vi "rsscope_core_global.vi"() -> ()   [LabVIEW 2018] (continued)
 parameter.  The trigger does not actually occur until the edge of a pulse that corresponds to the Glitch Width and Glitch Polarity crosses the threshold you specify in the Trigger Level parameter."}, {"Level"=4, "Class Only"=FALSE, "Identifier"="RSSCOPE_ATTR_SEARCH_TRIGGER_GLITCH_ENABLED", "Descriptive Name"="Search Trigger Glitch Enabled", "Data Type"=3, "Command"="SEAR:TRIG:GLIT", "Access"=2, "Range Table"="", "Read Callback"="rsscope_FormatSearchNameBoolean_ReadCallback.vi", "Write Callback"="rsscope_FormatSearchNameBoolean_WriteCallback.vi", "Supported Models"="", "Instrument Options"="", "Flags"=0, "Help"="Includes the search conditions for the glitch trigger event type in the next search.\n\nAvailable Repeated Capabilities:\nNone\n\nRemote-control command(s):\nSEARch:TRIGger:GLITch[:STATe]"}, {"Level"=4, "Class Only"=FALSE, "Identifier"="RSSCOPE_ATTR_SEARCH_TRIGGER_GLITCH_WIDTH", "Descriptive Name"="Search Trigger Glitch Width", "Data Type"=1, "Command"="SEAR:TRIG:GLIT:WIDT", "Access"=2, "Range Table"="RsScope_rngSearchGlitchWidth", "Read Callback"="rsscope_FormatSearchNameReal64_ReadCallback.vi", "Write Callback"="rsscope_FormatSearchNameReal64_WriteCallback.vi", "Supported Models"="", "Instrument Options"="", "Flags"=0, "Help"="Sets the length of a glitch. The instrument triggers on pulses shorter or longer than this value.\n\nAvailable Repeated Capabilities:\nNone\n\nRemote-control command(s):\nSEARch:TRIGger:GLITch:WIDTh"}, {"Level"=4, "Class Only"=FALSE, "Identifier"="RSSCOPE_ATTR_SEARCH_TRIGGER_GLITCH_POLARITY", "Descriptive Name"="Search Trigger Glitch Polarity", "Data Type"=0, "Command"="SEAR:TRIG:GLIT:POL", "Access"=2, "Range Table"="rsscope_rngTriggerSlope", "Read Callback"="rsscope_FormatSearchNameInt32_ReadCallback.vi", "Write Callback"="rsscope_FormatSearchNameInt32_WriteCallback.vi", "Supported Models"="", "Instrument Options"="", "Flags"=0, "Help"="Defines the polarity of a pulse, that is the direction of the first pulse slope.\n\nAvailable Repeated Capabilities:\nNone\n\nRemote-control command(s):\nSEARch:TRIGger:GLITch:POLarity"}, {"Level"=4, "Class Only"=FALSE, "Identifier"="RSSCOPE_ATTR_SEARCH_TRIGGER_GLITCH_CONDITION", "Descriptive Name"="Search Trigger Glitch Condition", "Data Type"=0, "Command"="SEAR:TRIG:GLIT:RANG", "Access"=2, "Range Table"="rsscope_rngWidthCondition", "Read Callback"="rsscope_FormatSearchNameInt32_ReadCallback.vi", "Write Callback"="rsscope_FormatSearchNameInt32_WriteCallback.vi", "Supported Models"="", "Instrument Options"="", "Flags"=0, "Help"="Selects which glitches are identified: shorter or longer than the specified width.\n\nAvailable Repeated Capabilities:\nNone\n\nRemote-control command(s):\nSEARch:TRIGger:GLITch:RANGe"}, {"Level"=4, "Class Only"=FALSE, "Identifier"="RSSCOPE_ATTR_SEARCH_TRIGGER_GLITCH_COPY_FROM_A", "Descriptive Name"="Search Trigger Glitch Copy From A", "Data Type"=4, "Command"="SEAR:TRIG:GLIT:ACOP", "Access"=1, "Range Table"="", "Read Callback"="", "Write Callback"="rsscope_FormatSearchNameEvent_WriteCallback.vi", "Supported Models"="", "Instrument Options"="", "Flags"=0, "Help"="Copies the trigger event configuration from Trigger A for the selected channel source to the search condition settings. Set the selected search name with RSSCOPE_ATTR_SELECTED_SEARCH_NAME.\n\nAvailable Repeated Capabilities:\nNone\n\nRemote-control command(s):\nSEARch:TRIGger:GLITch:ACOPy"}, {"Level"=3, "Class Only"=TRUE, "Identifier"="", "Descriptive Name"="Width", "Data Type"=0, "Command"="", "Access"=0, "Range Table"="", "Read Callback"="", "Write Callback"="", "Supported Models"="", "Instrument Options"="", "Flags"=0, "Help"="Configures the conditions for the width trigger search.  A width trigger occurs when the oscilloscope detects a positive or negative pulse with a width between, or optionally outside, the width thresholds.  You specify the width thresholds with the Width Low Threshold and Width High Threshold parameters.  You specify whether the oscilloscope triggers on pulse widths that are within or outside the width thresholds with the Width Condition parameter.  You specify the polarity of the pulse with the Width Polarity parameter.  The trigger does not actually occur until the edge of a pulse that corresponds to the Width Low Threshold, Width High Threshold, Width Condition, and Width Polarity crosses the threshold you specify in the Trigger Level parameter."}, {"Level"=4, "Class Only"=FALSE, "Identifier"="RSSCOPE_ATTR_SEARCH_TRIGGER_WIDTH_ENABLED", "Descriptive Name"="Search Trigger Width Enabled", "Data Type"=3, "Command"="SEAR:TRIG:WIDT", "Access"=2, "Range Table"="", "Read Callback"="rsscope_FormatSearchNameBoolean_ReadCallback.vi", "Write Callback"="rsscope_FormatSearchNameBoolean_WriteCallback.vi", "Supported Models"="", "Instrument Options"="", "Flags"=0, "Help"="Includes the search conditions for the width trigger event type in the next search.\n\nAvailable Repeated Capabilities:\nNone\n\nRemote-control command(s):\nSEARch:TRIGger:WIDTh[:STATe]"}, {"Level"=4, "Class Only"=FALSE, "Identifier"="RSSCOPE_ATTR_SEARCH_TRIGGER_WIDTH", "Descriptive Name"="Search Trigger Width", "Data Type"=1, "Command"="SEAR:TRIG:WIDT:WIDT", "Access"=2, "Range Table"="RsScope_rngSearchTriggerWidth", "Read Callback"="rsscope_FormatSearchNameReal64_ReadCallback.vi", "Write Callback"="rsscope_FormatSearchNameReal64_WriteCallback.vi", "Supported Models"="", "Instrument Options"="", "Flags"=0, "Help"="For the ranges &apos;Within&apos; and &apos;Outside&apos;, the width defines the center of a range which is defined by the limits &apos;+/-Delta&apos;. For the ranges &apos;Shorter&apos; and &apos;Longer&apos;, the width defines the maximum and minimum pulse width, respectively.\n\nAvailable Repeated Capabilities:\nNone\n\nRemote-control command(s):\nSEARch:TRIGger:WIDTh:WIDTh"}, {"Level"=4, "Class Only"=FALSE, "Identifier"="RSSCOPE_ATTR_SEARCH_TRIGGER_WIDTH_DELTA", "Descriptive Name"="Search Trigger Width Delta", "Data Type"=1, "Command"="SEAR:TRIG:WIDT:DELT", "Access"=2, "Range Table"="RsScope_rngSearchTriggerDelta", "Read Callback"="rsscope_FormatSearchNameReal64_ReadCallback.vi", "Write Callback"="rsscope_FormatSearchNameReal64_WriteCallback.vi", "Supported Models"="", "Instrument Options"="", "Flags"=0, "Help"="fines a range around the width value.\n\nAvailable Repeated Capabilities:\nNone\n\nRemote-control command(s):\nSEARch:TRIGger:WIDTh:DELTa"}, {"Level"=4, "Class Only"=FALSE, "Identifier"="RSSCOPE_ATTR_SEARCH_TRIGGER_WIDTH_POLARITY", "Descriptive Name"="Search Trigger Width Polarity", "Data Type"=0, "Command"="SEAR:TRIG:WIDT:POL", "Access"=2, "Range Table"="rsscope_rngTriggerSlope", "Read Callback"="rsscope_FormatSearchNameInt32_ReadCallback.vi", "Write Callback"="rsscope_FormatSearchNameInt32_WriteCallback.vi", "Supported Models"="", "Instrument Options"="", "Flags"=0, "Help"="Sets the polarity of the pulse.\n\nAvailable Repeated Capabilities:\nNone\n\nRemote-control command(s):\nSEARch:TRIGger:WIDTh:POLarity"}, {"Level"=4, "Class Only"=FALSE, "Identifier"="RSSCOPE_ATTR_SEARCH_TRIGGER_WIDTH_RANGE", "Descriptive Name"="Search Trigger Width Range", "Data Type"=0, "Command"="SEAR:TRIG:WIDT:RANG", "Access"=2, "Range Table"="rsscope_rngWidthCondition", "Read Callback"="rsscope_FormatSearchNameInt32_ReadCallback.vi", "Write Callback"="rsscope_FormatSearchNameInt32_WriteCallback.vi", "Supported Models"="", "Instrument Options"="", "Flags"=0, "Help"="Sets how the measured pulse width is compared with the given limit(s).\n\nAvailable Repeated Capabilities:\nNone\n\nRemote-control command(s):\nSEARch:TRIGger:WIDTh:RANGe"}, {"Level"=4, "Class Only"=FALSE, "Identifier"="RSSCOPE_ATTR_SEARCH_TRIGGER_WIDTH_COPY_FROM_A", "Descriptive Name"="Search Trigger Width Copy From A", "Data Type"=4, "Command"="SEAR:TRIG:WIDT:ACOP", "Access"=1, "Range Table"="", "Read Callback"="", "Write Callback"="rsscope_FormatSearchNameEvent_WriteCallback.vi", "Supported Models"="", "Instrument Options"="", "Flags"=0, "Help"="Copies the trigger event configuration from Trigger A for the selected channel source to the search condition settings. Set the selected search name with RSSCOPE_ATTR_SELECTED_SEARCH_NAME.\n\nAvailable Repeated Capabilities:\nNone\n\nRemote-control command(s):\nSEARch:TRIGger:WIDTh:ACOPy"}, {"Level"=3, "Class Only"=TRUE, "Identifier"="", "Descriptive Name"="Runt", "Data Type"=0, "Command"="", "Access"=0, "Range Table"="", "Read Callback"="", "Write Callback"="", "Supported Models"="", "Instrument Options"="", "Flags"=0, "Help"="This class configures the conditions for the runt trigger search. A runt trigger occurs when the trigger signal crosses one of the runt thresholds twice without crossing the other runt threshold.  You specify the runt thresholds with the  Runt Low Threshold and Runt High Threshold parameters.  You specify the polarity of the runt with the Runt Polarity parameter."}, {"Level"=4, "Class Only"=FALSE, "Identifier"="RSSCOPE_ATTR_SEARCH_TRIGGER_RUNT_ENABLED", "Descriptive Name"="Search Trigger Runt Enabled", "Data Type"=3, "Command"="SEAR:TRIG:RUNT", "Access"=2, "Range Table"="", "Read Callback"="rsscope_FormatSearchNameBoolean_ReadCallback.vi", "Write Callback"="rsscope_FormatSearchNameBoolean_WriteCallback.vi", "Supported Models"="", "Instrument Options"="", "Flags"=0, "Help"="Includes the search conditions for the runt trigger event type in the next search.\n\nAvailable Repeated Capabilities:\nNone\n\nRemote-control command(s):\nSEARch:TRIGger:RUNT[:STATe]"}, {"Level"=4, "Class Only"=FALSE, "Identifier"="RSSCOPE_ATTR_SEARCH_TRIGGER_RUNT_UPPER_LEVEL", "Descriptive Name"="Search Trigger Runt Upper Level", "Data Type"=1, "Command"="SEAR:TRIG:LEV:RUNT:UPP", "Access"=2, "Range Table"="", "Read Callback"="rsscope_FormatSearchNameSourceReal64_ReadCallback.vi", "Write Callback"="rsscope_FormatSearchNameSourceReal64_WriteCallback.vi", "Supported Models"="", "Instrument Options"="", "Flags"=0, "Help"="Set the upper voltage threshold.\n\nAvailable Repeated Capabilities:\nNone\n\nRemote-control command(s):\nSEARch:TRIGger:LEVel:RUNT:UPPer"}, {"Level"=4, "Class Only"=FALSE, "Identifier"="RSSCOPE_ATTR_SEARCH_TRIGGER_RUNT_LOWER_LEVEL", "Descriptive Name"="Search Trigger Runt Lower Level", "Data Type"=1, "Command"="SEAR:TRIG:LEV:RUNT:LOW", "Access"=2, "Range Table"="", "Read Callback"="rsscope_FormatSearchNameSourceReal64_ReadCallback.vi", "Write Callback"="rsscope_FormatSearchNameSourceReal64_WriteCallback.vi", "Supported Models"="", "Instrument Options"="", "Flags"=0, "Help"="Set the lower voltage threshold.\n\nAvailable Repeated Capabilities:\nNone\n\nRemote-control command(s):\nSEARch:TRIGger:LEVel:RUNT:LOWer"}, {"Level"=4, "Class Only"=FALSE, "Identifier"="RSSCOPE_ATTR_SEARCH_TRIGGER_RUNT_POLARITY", "Descriptive Name"="Search Trigger Runt Polarity", "Data Type"=0, "Command"="SEAR:TRIG:RUNT:POL", "Access"=2, "Range Table"="rsscope_rngTriggerSlope", "Read Callback"="rsscope_FormatSearchNameInt32_ReadCallback.vi", "Write Callback"="rsscope_FormatSearchNameInt32_WriteCallback.vi", "Supported Models"="", "Instrument Options"="", "Flags"=0, "Help"="Defines the polarity of a pulse, that is the direction of the first pulse slope.\n\nAvailable Repeated Capabilities:\nNone\n\nRemote-control command(s):\nSEARch:TRIGger:RUNT:POLarity"}, {"Level"=4, "Class Only"=FALSE, "Identifier"="RSSCOPE_ATTR_SEARCH_TRIGGER_RUNT_WIDTH", "Descriptive Name"="Search Trigger Runt Width", "Data Type"=1, "Command"="SEAR:TRIG:RUNT:WIDT", "Access"=2, "Range Table"="RsScope_rngSearchTriggerWidth", "Read Callback"="rsscope_FormatSearchNameReal64_ReadCallback.vi", "Write Callback"="rsscope_FormatSearchNameReal64_WriteCallback.vi", "Supported Models"="", "Instrument Options"="", "Flags"=0, "Help"="For the ranges &apos;Shorter&apos; and &apos;Longer&apos;, the runt width defines the maximum and minimum pulse width, respectively.\nFor the ranges &apos;Within&apos; and &apos;Outside&apos;, the runt width defines the center of a range which is defined by &apos;+/-Delta&apos;.\n\nAvailable Repeated Capabilities:\nNone\n\nRemote-control command(s):\nSEARch:TRIGger:RUNT:WIDTh"}, {"Level"=4, "Class Only"=FALSE, "Identifier"="RSSCOPE_ATTR_SEARCH_TRIGGER_RUNT_DELTA", "Descriptive Name"="Search Trigger Runt Delta", "Data Type"=1, "Command"="SEAR:TRIG:RUNT:DELT", "Access"=2, "Range Table"="RsScope_rngSearchTriggerRuntDelta", "Read Callback"="rsscope_FormatSearchNameReal64_ReadCallback.vi", "Write Callback"="rsscope_FormatSearchNameReal64_WriteCallback.vi", "Supported Models"="", "Instrument Options"="", "Flags"=0, "Help"="Defines a range around the runt width specified using Runt Width.\n\nAvailable Repeated Capabilities:\nNone\n\nRemote-control command(s):\nSEARch:TRIGger:RUNT:DELTa"}, {"Level"=4, "Class Only"=FALSE, "Identifier"="RSSCOPE_ATTR_SEARCH_TRIGGER_RUNT_RANGE", "Descriptive Name"="Search Trigger Runt Range", "Data Type"=0, "Command"="SEAR:TRIG:RUNT:RANG", "Access"=2, "Range Table"="RsScope_rngSearchTriggerRuntRange", "Read Callback"="rsscope_FormatSearchNameInt32_ReadCallback.vi", "Write Callback"="rsscope_FormatSearchNameInt32_WriteCallback.vi", "Supported Models"="", "Instrument Options"="", "Flags"=0, "Help"="Selects how the time limit of the runt pulse is defined based on the runt width and delta\n\nAvailable Repeated Capabilities:\nNone\n\nRemote-control command(s):\nSEARch:TRIGger:RUNT:RANGe"}, {"Level"=4, "Class Only"=FALSE, "Identifier"="RSSCOPE_ATTR_SEARCH_TRIGGER_RUNT_COPY_FROM_A", "Descriptive Name"="Search Trigger Runt Copy From A", "Data Type"=4, "Command"="SEAR:TRIG:RUNT:ACOP", "Access"=1, "Range Table"="", "Read Callback"="", "Write Callback"="rsscope_FormatSearchNameEvent_WriteCallback.vi", "Supported Models"="", "Instrument Options"="", "Flags"=0, "Help"="Copies the trigger event configuration from Trigger A for the selected channel source to the search condition settings. Set the selected search name with RSSCOPE_ATTR_SELECTED_SEARCH_NAME.\n\nAvailable Repeated Capabilities:\nNone\n\nRemote-control command(s):\nSEARch:TRIGger:RUNT:ACOPy"}, {"Level"=3, "Class Only"=TRUE, "Identifier"="", "Descriptive Name"="Window", "Data Type"=0, "Command"="", "Access"=0, "Range Table"="", "Read Callback"="", "Write Callback"="", "Supported Models"="", "Instrument Options"="", "Flags"=0, "Help"="This class configures the conditions for the window trigger search. The window trigger checks the signal run in relation to a &apos;window&apos;. The window is formed by the upper and lower voltage levels. The event condition is fulfilled, if the waveform enters or leaves the window, or if the waveform stays inside or outside for a time longer or shorter than specified. With the window trigger, you can display longer transient effects."}, {"Level"=4, "Class Only"=FALSE, "Identifier"="RSSCOPE_ATTR_SEARCH_TRIGGER_WINDOW_ENABLED", "Descriptive Name"="Search Trigger Window Enabled", "Data Type"=3, "Command"="SEAR:TRIG:WIND", "Access"=2, "Range Table"="", "Read Callback"="rsscope_FormatSearchNameBoolean_ReadCallback.vi", "Write Callback"="rsscope_FormatSearchNameBoolean_WriteCallback.vi", "Supported Models"="", "Instrument Options"="", "Flags"=0, "Help"="Includes the search conditions for the window trigger event type in the next search.\n\nAvailable Repeated Capabilities:\nNone\n\nRemote-control command(s):\nSEARch:TRIGger:WINDow[:STATe]"}, {"Level"=4, "Class Only"=FALSE, "Identifier"="RSSCOPE_ATTR_SEARCH_TRIGGER_WINDOW_UPPER_LEVEL", "Descriptive Name"="Search Trigger Window Upper Level", "Data Type"=1, "Command"="SEAR:TRIG:LEV:WIND:UPP", "Access"=2, "Range Table"="", "Read Callback"="rsscope_FormatSearchNameSourceReal64_ReadCallback.vi", "Write Callback"="rsscope_FormatSearchNameSourceReal64_WriteCallback.vi", "Supported Models"="", "Instrument Options"="", "Flags"=0, "Help"="Set the upper voltage threshold.\n\nAvailable Repeated Capabilities:\nNone\n\nRemote-control command(s):\nSEARch:TRIGger:LEVel:WINDow:UPPer"}, {"Level"=4, "Class Only"=FALSE, "Identifier"="RSSCOPE_ATTR_SEARCH_TRIGGER_WINDOW_LOWER_LEVEL", "Descriptive Name"="Search Trigger Window Lower Level", "Data Type"=1, "Command"="SEAR:TRIG:LEV:WIND:LOW", "Access"=2, "Range Table"="", "Read Callback"="rsscope_FormatSearchNameSourceReal64_ReadCallback.vi", "Write Callback"="rsscope_FormatSearchNameSourceReal64_WriteCallback.vi", "Supported Models"="", "Instrument Options"="", "Flags"=0, "Help"="Set the lower voltage threshold.\n\nAvailable Repeated Capabilities:\nNone\n\nRemote-control command(s):\nSEARch:TRIGger:LEVel:WINDow:LOWer"}, {"Level"=4, "Class Only"=FALSE, "Identifier"="RSSCOPE_ATTR_SEARCH_TRIGGER_WINDOW_VERTICAL_CONDITION", "Descriptive Name"="Search Trigger Window Vertical Condition", "Data Type"=0, "Command"="SEAR:TRIG:WIND:RANG", "Access"=2, "Range Table"="RsScope_rngSearchTriggerWindowVerticalCondition", "Read Callback"="rsscope_FormatSearchNameInt32_ReadCallback.vi", "Write Callback"="rsscope_FormatSearchNameInt32_WriteCallback.vi", "Supported Models"="", "Instrument Options"="", "Flags"=0, "Help"="Defines the signal run in relation to the window.\n\nAvailable Repeated Capabilities:\nNone\n\nRemote-control command(s):\nSEARch:TRIGger:WINDow:RANGe"}, {"Level"=4, "Class Only"=FALSE, "Identifier"="RSSCOPE_ATTR_SEARCH_TRIGGER_WINDOW_TIME_CONDITION", "Descriptive Name"="Search Trigger Window Time Condition", "Data Type"=0, "Command"="SEAR:TRIG:WIND:TIM", "Access"=2, "Range Table"="rsscope_rngWidthCondition", "Read Callback"="rsscope_FormatSearchNameInt32_ReadCallback.vi", "Write Callback"="rsscope_FormatSearchNameInt32_WriteCallback.vi", "Supported Models"="", "Instrument Options"="", "Flags"=0, "Help"="Selects how the time limit of the window is defined. Time conditioning is available for the vertical conditions &apos;WITHin&apos; and &apos;OUTSide&apos;.\n\nAvailable Repeated Capabilities:\nNone\n\nRemote-control command(s):\nSEARch:TRIGger:WINDow:TIMerange"}, {"Level"=4, "Class Only"=FALSE, "Identifier"="RSSCOPE_ATTR_SEARCH_TRIGGER_WINDOW_WIDTH", "Descriptive Name"="Search Trigger Window Width", "Data Type"=1, "Command"="SEAR:TRIG:WIND:WIDT", "Access"=2, "Range Table"="RsScope_rngSearchTriggerWidth", "Read Callback"="rsscope_FormatSearchNameReal64_ReadCallback.vi", "Write Callback"="rsscope_FormatSearchNameReal64_WriteCallback.vi", "Supported Models"="", "Instrument Options"="", "Flags"=0, "Help"="For the ranges &apos;Shorter&apos; and &apos;Longer&apos;, the runt width defines the maximum and minimum pulse width, respectively.\nFor the ranges &apos;Within&apos; and &apos;Outside&apos;, the runt width defines the center of a range which is defined by &apos;+/-Delta&apos;.\n\nAvailable Repeated Capabilities:\nNone\n\nRemote-control command(s):\nSEARch:TRIGger:WINDow:WIDTh"}, {"Level"=4, "Class Only"=FALSE, "Identifier"="RSSCOPE_ATTR_SEARCH_TRIGGER_WINDOW_DELTA", "Descriptive Name"="Search Trigger Window Delta", "Data Type"=1, "Command"="SEAR:TRIG:WIND:DELT", "Access"=2, "Range Table"="RsScope_rngSearchTriggerDelta", "Read Callback"="rsscope_FormatSearchNameReal64_ReadCallback.vi", "Write Callback"="rsscope_FormatSearchNameReal64_WriteCallback.vi", "Supported Models"="", "Instrument Options"="", "Flags"=0, "Help"="Defines a range around the width value.\n\nAvailable Repeated Capabilities:\nNone\n\nRemote-control command(s):\nSEARch:TRIGger:WINDow:DELTa"}, {"Level"=4, "Class Only"=FALSE, "Identifier"="RSSCOPE_ATTR_SEARCH_TRIGGER_WINDOW_COPY_FROM_A", "Descriptive Name"="Search Trigger Window Copy From A", "Data Type"=4, "Command"="SEAR:TRIG:WIND:ACOP", "Access"=1, "Range Table"="", "Read Callback"="", "Write Callback"="rsscope_FormatSearchNameEvent_WriteCallback.vi", "Supported Models"="", "Instrument Options"="", "Flags"=0, "Help"="Copies the trigger event configuration from Trigger A for the selected channel source to the search condition settings. Set the selected search name with RSSCOPE_ATTR_SELECTED_SEARCH_NAME.\n\nAvailable Repeated Capabilities:\nNone\n\nRemote-control command(s):\nSEARch:TRIGger:WINDow:ACOPy"}, {"Level"=3, "Class Only"=TRUE, "Identifier"="", "Descriptive Name"="Timeout", "Data Type"=0, "Command"="", "Access"=0, "Range Table"="", "Read Callback"="", "Write Callback"="", "Supported Models"="", "Instrument Options"="", "Flags"=0, "Help"="This class configures the conditions for the timeout trigger search. The timeout trigger event checks if the signal stays above or below the threshold voltage for a specified time lapse. In other words, the event occurs if the trigger source does not have the expected transition within the specified time."}, {"Level"=4, "Class Only"=FALSE, "Identifier"="RSSCOPE_ATTR_SEARCH_TRIGGER_TIMEOUT_ENABLED", "Descriptive Name"="Search Trigger Timeout Enabled", "Data Type"=3, "Command"="SEAR:TRIG:TIM", "Access"=2, "Range Table"="", "Read Callback"="rsscope_FormatSearchNameBoolean_ReadCallback.vi", "Write Callback"="rsscope_FormatSearchNameBoolean_WriteCallback.vi", "Supported Models"="", "Instrument Options"="", "Flags"=0, "Help"="Includes the search conditions for the timeout trigger event type in the next search.\n\nAvailable Repeated Capabilities:\nNone\n\nRemote-control command(s):\nSEARch:TRIGger:TIMeout[:STATe]"}, {"Level"=4, "Class Only"=FALSE, "Identifier"="RSSCOPE_ATTR_SEARCH_TRIGGER_TIMEOUT_VALUE", "Descriptive Name"="Search Trigger Timeout Value", "Data Type"=1, "Command"="SEAR:TRIG:TIM:TIME", "Access"=2, "Range Table"="RsScope_rngSearchTriggerWidth", "Read Callback"="rsscope_FormatSearchNameReal64_ReadCallback.vi", "Write Callback"="rsscope_FormatSearchNameReal64_WriteCallback.vi", "Supported Models"="", "Instrument Options"="", "Flags"=0, "Help"="Defines the time limit for the timeout at which the instrument triggers.\n\nAvailable Repeated Capabilities:\nNone\n\nRemote-control command(s):\nSEARch:TRIGger:TIMeout:TIME"}, {"Level"=4, "Class Only"=FALSE, "Identifier"="RSSCOPE_ATTR_SEARCH_TRIGGER_TIMEOUT_CONDITION", "Descriptive Name"="Search Trigger Timeout Condition", "Data Type"=0, "Command"="SEAR:TRIG:TIM:RANG", "Access"=2, "Range Table"="RsScope_rngSearchTriggerTimeoutCondition", "Read Callback"="rsscope_FormatSearchNameInt32_ReadCallback.vi", "Write Callback"="rsscope_FormatSearchNameInt32_WriteCallback.vi", "Supported Models"="", "Instrument Options"="", "Flags"=0, "Help"="Defines the relation of the signal level to the trigger level.\n\nAvailable Repeated Capabilities:\nNone\n\nRemote-control command(s):\nSEARch:TRIGger:TIMeout:RANGe"}, {"Level"=4, "Class Only"=FALSE, "Identifier"="RSSCOPE_ATTR_SEARCH_TRIGGER_TIMEOUT_COPY_FROM_A", "Descriptive Name"="Search Trigger Timeout Copy From A", "Data Type"=4, "Command"="SEAR:TRIG:TIM:ACOP", "Access"=1, "Range Table"="", "Read Callback"="", "Write Callback"="rsscope_FormatSearchNameEvent_WriteCallback.vi", "Supported Models"="", "Instrument Options"="", "Flags"=0, "Help"="Copies the trigger event configuration from Trigger A for the selected channel source to the search condition settings. Set the selected search name with RSSCOPE_ATTR_SELECTED_SEARCH_NAME.\n\nAvailable Repeated Capabilities:\nNone\n\nRemote-control command(s):\nSEARch:TRIGger:TIMeout:ACOPy"}, {"Level"=3, "Class Only"=TRUE, "Identifier"="", "Descriptive Name"="Interval", "Data Type"=0, "Command"="", "Access"=0, "Range Table"="", "Read Callback"="", "Write Callback"="", "Supported Models"="", "Instrument Options"="", "Flags"=0, "Help"="This class configures the conditions for the interval trigger search. The interval trigger analyzes the time between two pulses. While the interval trigger can only analyze either positive or negative polarity, searching for an interval is also possible for both polarities at the same time (&apos;Either&apos;)."}, {"Level"=4, "Class Only"=FALSE, "Identifier"="RSSCOPE_ATTR_SEARCH_TRIGGER_INTERVAL_ENABLED", "Descriptive Name"="Search Trigger Interval Enabled", "Data Type"=3, "Command"="SEAR:TRIG:INT", "Access"=2, "Range Table"="", "Read Callback"="rsscope_FormatSearchNameBoolean_ReadCallback.vi", "Write Callback"="rsscope_FormatSearchNameBoolean_WriteCallback.vi", "Supported Models"="", "Instrument Options"="", "Flags"=0, "Help"="Includes the search conditions for the interval trigger event type in the next search.\n\nAvailable Repeated Capabilities:\nNone\n\nRemote-control command(s):\nSEARch:TRIGger:INTerval[:STATe]"}, {"Level"=4, "Class Only"=FALSE, "Identifier"="RSSCOPE_ATTR_SEARCH_TRIGGER_INTERVAL_WIDTH", "Descriptive Name"="Search Trigger Interval Width", "Data Type"=1, "Command"="SEAR:TRIG:INT:WIDT", "Access"=2, "Range Table"="RsScope_rngSearchTriggerIntervalWidth", "Read Callback"="rsscope_FormatSearchNameReal64_ReadCallback.vi", "Write Callback"="rsscope_FormatSearchNameReal64_WriteCallback.vi", "Supported Models"="", "Instrument Options"="", "Flags"=0, "Help"="Defines the time between two pulses\n\nAvailable Repeated Capabilities:\nNone\n\nRemote-control command(s):\nSEARch:TRIGger:INTerval:WIDTh"}, {"Level"=4, "Class Only"=FALSE, "Identifier"="RSSCOPE_ATTR_SEARCH_TRIGGER_INTERVAL_DELTA", "Descriptive Name"="Search Trigger Interval Delta", "Data Type"=1, "Command"="SEAR:TRIG:INT:DELT", "Access"=2, "Range Table"="RsScope_rngSearchTriggerIntervalDelta", "Read Callback"="rsscope_FormatSearchNameReal64_ReadCallback.vi", "Write Callback"="rsscope_FormatSearchNameReal64_WriteCallback.vi", "Supported Models"="", "Instrument Options"="", "Flags"=0, "Help"="Defines a range around the &apos;Interval width&apos; value.\n\nAvailable Repeated Capabilities:\nNone\n\nRemote-control command(s):\nSEARch:TRIGger:INTerval:DELTa"}, {"Level"=4, "Class Only"=FALSE, "Identifier"="RSSCOPE_ATTR_SEARCH_TRIGGER_INTERVAL_POLARITY", "Descriptive Name"="Search Trigger Interval Polarity", "Data Type"=0, "Command"="SEAR:TRIG:INT:SLOP", "Access"=2, "Range Table"="rsscope_rngTriggerSlope", "Read Callback"="rsscope_FormatSearchNameInt32_ReadCallback.vi", "Write Callback"="rsscope_FormatSearchNameInt32_WriteCallback.vi", "Supported Models"="", "Instrument Options"="", "Flags"=0, "Help"="Sets the polarity of the pulse.\n\nAvailable Repeated Capabilities:\nNone\n\nRemote-control command(s):\nSEARch:TRIGger:INTerval:SLOPe"}, {"Level"=4, "Class Only"=FALSE, "Identifier"="RSSCOPE_ATTR_SEARCH_TRIGGER_INTERVAL_CONDITION", "Descriptive Name"="Search Trigger Interval Condition", "Data Type"=0, "Command"="SEAR:TRIG:INT:RANG", "Access"=2, "Range Table"="rsscope_rngWidthCondition", "Read Callback"="rsscope_FormatSearchNameInt32_ReadCallback.vi", "Write Callback"="rsscope_FormatSearchNameInt32_WriteCallback.vi", "Supported Models"="", "Instrument Options"="", "Flags"=0, "Help"="Defines the range of an interval in relation to the interval width.\n\nAvailable Repeated Capabilities:\nNone\n\nRemote-control command(s):\nSEARch:TRIGger:INTerval:RANGe"}, {"Level"=4, "Class Only"=FALSE, "Identifier"="RSSCOPE_ATTR_SEARCH_TRIGGER_INTERVAL_COPY_FROM_A", "Descriptive Name"="Search Trigger Interval Copy From A", "Data Type"=4, "Command"="SEAR:TRIG:INT:ACOP", "Access"=1, "Range Table"="", "Read Callback"="", "Write Callback"="rsscope_FormatSearchNameEvent_WriteCallback.vi", "Supported Models"="", "Instrument Options"="", "Flags"=0, "Help"="Copies the trigger event configuration from Trigger A for the selected channel source to the search condition settings. Set the selected search name with RSSCOPE_ATTR_SELECTED_SEARCH_NAME.\n\nAvailable Repeated Capabilities:\nNone\n\nRemote-control command(s):\nSEARch:TRIGger:INTerval:ACOPy"}, {"Level"=3, "Class Only"=TRUE, "Identifier"="", "Descriptive Name"="Slew Rate", "Data Type"=0, "Command"="", "Access"=0, "Range Table"="", "Read Callback"="", "Write Callback"="", "Supported Models"="", "Instrument Options"="", "Flags"=0, "Help"="This class configures the conditions for the slew rate trigger search. The slew rate trigger, also known as transition trigger, can detect fast or slow edges selectively. It triggers on edges, if the transition time from the lower to higher voltage level (or vice versa) is shorter or longer as defined, or outside a specified time range. The trigger event finds slew rates faster than expected or permissible to avoid overshooting and other interfering effects. It also detects very slow edges violating the timing in pulse series."}, {"Level"=4, "Class Only"=FALSE, "Identifier"="RSSCOPE_ATTR_SEARCH_TRIGGER_SLEW_RATE_ENABLED", "Descriptive Name"="Search Trigger Slew Rate Enabled", "Data Type"=3, "Command"="SEAR:TRIG:SLEW", "Access"=2, "Range Table"="", "Read Callback"="rsscope_FormatSearchNameBoolean_ReadCallback.vi", "Write Callback"="rsscope_FormatSearchNameBoolean_WriteCallback.vi", "Supported Models"="", "Instrument Options"="", "Flags"=0, "Help"="Includes the search conditions for the slew rate trigger event type in the next search.\n\nAvailable Repeated Capabilities:\nNone\n\nRemote-control command(s):\nSEARch:TRIGger:SLEWrate[:STATe]"}, {"Level"=4, "Class Only"=FALSE, "Identifier"="RSSCOPE_ATTR_SEARCH_TRIGGER_SLEW_RATE_UPPER_LEVEL", "Descriptive Name"="Search Trigger Slew Rate Upper Level", "Data Type"=1, "Command"="SEAR:TRIG:LEV:TRAN:UPP", "Access"=2, "Range Table"="", "Read Callback"="rsscope_FormatSearchNameSourceReal64_ReadCallback.vi", "Write Callback"="rsscope_FormatSearchNameSourceReal64_WriteCallback.vi", "Supported Models"="", "Instrument Options"="", "Flags"=0, "Help"="Set the upper voltage threshold.\n\nAvailable Repeated Capabilities:\nNone\n\nRemote-control command(s):\nSEARch:TRIGger:LEVel:TRANsition:UPPer"}, {"Level"=4, "Class Only"=FALSE, "Identifier"="RSSCOPE_ATTR_SEARCH_TRIGGER_SLEW_RATE_LOWER_LEVEL", "Descriptive Name"="Search Trigger Slew Rate Lower Level", "Data Type"=1, "Command"="SEAR:TRIG:LEV:TRAN:LOW", "Access"=2, "Range Table"="", "Read Callback"="rsscope_FormatSearchNameSourceReal64_ReadCallback.vi", "Write Callback"="rsscope_FormatSearchNameSourceReal64_WriteCallback.vi", "Supported Models"="", "Instrument Options"="", "Flags"=0, "Help"="Set the lower voltage threshold.\n\nAvailable Repeated Capabilities:\nNone\n\nRemote-control command(s):\nSEARch:TRIGger:LEVel:TRANsition:LOWer"}, {"Level"=4, "Class Only"=FALSE, "Identifier"="RSSCOPE_ATTR_SEARCH_TRIGGER_SLEW_RATE_VALUE", "Descriptive Name"="Search Trigger Slew Rate Value", "Data Type"=1, "Command"="SEAR:TRIG:SLEW:TIME", "Access"=2, "Range Table"="RsScope_rngSearchTriggerWidth", "Read Callback"="rsscope_FormatSearchNameReal64_ReadCallback.vi", "Write Callback"="rsscope_FormatSearchNameReal64_WriteCallback.vi", "Supported Models"="", "Instrument Options"="", "Flags"=0, "Help"="For the ranges &apos;Within&apos; and &apos;Outside&apos;, the slew rate defines the center of a range which is defined by the limits &apos;Delta&apos;.\nFor the ranges &apos;Shorter&apos; and &apos;Longer&apos;, the slew rate defines the maximum and minimum slew rate limits, respectively. When the signal crosses this level, the slew rate measurement starts or stops depending on the selected slope.\n\nAvailable Repeated Capabilities:\nNone\n\nRemote-control command(s):\nSEARch:TRIGger:SLEWrate:TIME"}, {"Level"=4, "Class Only"=FALSE, "Identifier"="RSSCOPE_ATTR_SEARCH_TRIGGER_SLEW_RATE_DELTA", "Descriptive Name"="Search Trigger Slew Rate Delta", "Data Type"=1, "Command"="SEAR:TRIG:SLEW:DELT", "Access"=2, "Range Table"="RsScope_rngSearchTriggerIntervalDelta", "Read Callback"="rsscope_FormatSearchNameReal64_ReadCallback.vi", "Write Callback"="rsscope_FormatSearchNameReal64_WriteCallback.vi", "Supported Models"="", "Instrument Options"="", "Flags"=0, "Help"="Defines a range around the &apos;Interval width&apos; value.\n\nAvailable Repeated Capabilities:\nNone\n\nRemote-control command(s):\nSEARch:TRIGger:SLEWrate:DELTa"}, {"Level"=4, "Class Only"=FALSE, "Identifier"="RSSCOPE_ATTR_SEARCH_TRIGGER_SLEW_RATE_POLARITY", "Descriptive Name"="Search Trigger Slew Rate Polarity", "Data Type"=0, "Command"="SEAR:TRIG:SLEW:SLOP", "Access"=2, "Range Table"="rsscope_rngTriggerSlope", "Read Callback"="rsscope_FormatSearchNameInt32_ReadCallback.vi", "Write Callback"="rsscope_FormatSearchNameInt32_WriteCallback.vi", "Supported Models"="", "Instrument Options"="", "Flags"=0, "Help"="Defines the polarity of a pulse, that is the direction of the first pulse slope.\n\nAvailable Repeated Capabilities:\nNone\n\nRemote-control command(s):\nSEARch:TRIGger:SLEWrate:SLOPe"}, {"Level"=4, "Class Only"=FALSE, "Identifier"="RSSCOPE_ATTR_SEARCH_TRIGGER_SLEW_RATE_CONDITION", "Descriptive Name"="Search Trigger Slew Rate Condition", "Data Type"=0, "Command"="SEAR:TRIG:SLEW:RANG", "Access"=2, "Range Table"="rsscope_rngSlewCondition", "Read Callback"="rsscope_FormatSearchNameInt32_ReadCallback.vi", "Write Callback"="rsscope_FormatSearchNameInt32_WriteCallback.vi", "Supported Models"="", "Instrument Options"="", "Flags"=0, "Help"="Selects how the time limit for the slew rate is defined. The time measurement starts when the signal crosses the first trigger level - the upper or lower level depending on the selected slope - and stops when the signal crosses the second level.\n\nAvailable Repeated Capabilities:\nNone\n\nRemote-control command(s):\nSEARch:TRIGger:SLEWrate:RANGe"}, {"Level"=4, "Class Only"=FALSE, "Identifier"="RSSCOPE_ATTR_SEARCH_TRIGGER_SLEW_RATE_COPY_FROM_A", "Descriptive Name"="Search Trigger Slew Rate Copy From A", "Data Type"=4, "Command"="SEAR:TRIG:SLEW:ACOP", "Access"=1, "Range Table"="", "Read Callback"="", "Write Callback"="rsscope_FormatSearchNameEvent_WriteCallback.vi", "Supported Models"="", "Instrument Options"="", "Flags"=0, "Help"="Copies the trigger event configuration from Trigger A for the selected channel source to the search condition settings. Set the selected search name with RSSCOPE_ATTR_SELECTED_SEARCH_NAME.\n\nAvailable Repeated Capabilities:\nNone\n\nRemote-control command(s):\nSEARch:TRIGger:SLEWrate:ACOPy"}, {"Level"=3, "Class Only"=TRUE, "Identifier"="", "Descriptive Name"="Data2Clock", "Data Type"=0, "Command"="", "Access"=0, "Range Table"="", "Read Callback"="", "Write Callback"="", "Supported Models"="", "Instrument Options"="", "Flags"=0, "Help"="This class configures the conditions for the data 2 clock trigger search. With the Data2Clock event - also known as setup/hold - you can analyze the relative timing between two signals: a data signal and the synchronous clock signal. Many systems require, that the data signal must be steady for some time before and after the clock edge, for example, the data transmission on parallel interfaces. With this trigger type, you can also test the time correlation of sideband and inband signals. The event occurs if the data signal crosses the data level during the setup and hold time. The reference point for the time measurement is defined by clock level and clock edge."}, {"Level"=4, "Class Only"=FALSE, "Identifier"="RSSCOPE_ATTR_SEARCH_TRIGGER_DATA2CLOCK_ENABLED", "Descriptive Name"="Search Trigger Data2Clock Enabled", "Data Type"=3, "Command"="SEAR:TRIG:DAT", "Access"=2, "Range Table"="", "Read Callback"="rsscope_FormatSearchNameBoolean_ReadCallback.vi", "Write Callback"="rsscope_FormatSearchNameBoolean_WriteCallback.vi", "Supported Models"="", "Instrument Options"="", "Flags"=0, "Help"="Includes the search conditions for the data2clock trigger event type in the next search.\n\nAvailable Repeated Capabilities:\nNone\n\nRemote-control command(s):\nSEARch:TRIGger:SETHold[:STATe]"}, {"Level"=4, "Class Only"=FALSE, "Identifier"="RSSCOPE_ATTR_SEARCH_TRIGGER_DATA2CLOCK_SOURCE", "Descriptive Name"="Search Trigger Data2Clock Source", "Data Type"=0, "Command"="SEAR:TRIG:SETH:CSO", "Access"=2, "Range Table"="RsScope_rngSearchSource", "Read Callback"="rsscope_FormatSearchNameInt32_ReadCallback.vi", "Write Callback"="rsscope_FormatSearchNameInt32_WriteCallback.vi", "Supported Models"="", "Instrument Options"="", "Flags"=0, "Help"="Selects the waveform used for the clock signal.\n\nAvailable Repeated Capabilities:\nNone\n\nRemote-control command(s):\nSEARch:TRIGger:SETHold:CSOurce"}, {"Level"=4, "Class Only"=FALSE, "Identifier"="RSSCOPE_ATTR_SEARCH_TRIGGER_DATA2CLOCK_LEVEL", "Descriptive Name"="Search Trigger Data2Clock Level", "Data Type"=1, "Command"="SEAR:TRIG:SETH:CLEV", "Access"=2, "Range Table"="RsScope_rngSearchTriggerClockLevel", "Read Callback"="rsscope_FormatSearchNameReal64_ReadCallback.vi", "Write Callback"="rsscope_FormatSearchNameReal64_WriteCallback.vi", "Supported Models"="", "Instrument Options"="", "Flags"=0, "Help"="Sets the voltage level for the clock signal.\n\nAvailable Repeated Capabilities:\nNone\n\nRemote-control command(s):\nSEARch:TRIGger:SETHold:CLEVel"}, {"Level"=4, "Class Only"=FALSE, "Identifier"="RSSCOPE_ATTR_SEARCH_TRIGGER_DATA2CLOCK_HOLD_TIME", "Descriptive Name"="Search Trigger Data2Clock Hold Time", "Data Type"=1, "Command"="SEAR:TRIG:SETH:HTIM", "Access"=2, "Range Table"="RsScope_rngSearchTriggerData2ClockTime", "Read Callback"="rsscope_FormatSearchNameReal64_ReadCallback.vi", "Write Callback"="rsscope_FormatSearchNameReal64_WriteCallback.vi", "Supported Models"="", "Instrument Options"="", "Flags"=0, "Help"="Sets the minimum time after the clock edge while the data signal must stay steady above or below the data level. The hold time can be negative. In this case, the setup time is always positive. The setup/hold interval starts before the clock edge (setup time) and ends before the clock edge (hold time). If you change the negative hold time, the setup time is adjusted by the intrument.\n\nAvailable Repeated Capabilities:\nNone\n\nRemote-control command(s):\nSEARch:TRIGger:SETHold:HTIMe"}, {"Level"=4, "Class Only"=FALSE, "Identifier"="RSSCOPE_ATTR_SEARCH_TRIGGER_DATA2CLOCK_SETUP_TIME", "Descriptive Name"="Search Trigger Data2Clock Setup Time", "Data Type"=1, "Command"="SEAR:TRIG:SETH:STIM", "Access"=2, "Range Table"="RsScope_rngSearchTriggerData2ClockTime", "Read Callback"="rsscope_FormatSearchNameReal64_ReadCallback.vi", "Write Callback"="rsscope_FormatSearchNameReal64_WriteCallback.vi", "Supported Models"="", "Instrument Options"="", "Flags"=0, "Help"="Sets the minimum time before the clock edge while the data signal must stay steady above or below the data level. The setup time can be negative. In this case, the hold time is always positive. The setup/hold interval starts after the clock edge (setup time) and ends after the clock edge (hold time). If you change the negative setup time, the hold time is adjusted by the intrument.\n\nAvailable Repeated Capabilities:\nNone\n\nRemote-control command(s):\nSEARch:TRIGger:SETHold:STIMe"}, {"Level"=4, "Class Only"=FALSE, "Identifier"="RSSCOPE_ATTR_SEARCH_TRIGGER_DATA2CLOCK_EDGE", "Descriptive Name"="Search Trigger Data2Clock Edge", "Data Type"=0, "Command"="SEAR:TRIG:SETH:CEDG", "Access"=2, "Range Table"="rsscope_rngTriggerSlope", "Read Callback"="rsscope_FormatSearchNameInt32_ReadCallback.vi", "Write Callback"="rsscope_FormatSearchNameInt32_WriteCallback.vi", "Supported Models"="", "Instrument Options"="", "Flags"=0, "Help"="Sets the edge of the clock signal to define the time reference point for the setup and hold time.\n\nAvailable Repeated Capabilities:\nNone\n\nRemote-control command(s):\nSEARch:TRIGger:SETHold:CEDGe"}, {"Level"=4, "Class Only"=FALSE, "Identifier"="RSSCOPE_ATTR_SEARCH_TRIGGER_DATA2CLOCK_COPY_FROM_A", "Descriptive Name"="Search Trigger Data2Clock Copy From A", "Data Type"=4, "Command"="SEAR:TRIG:SETH:ACOP", "Access"=1, "Range Table"="", "Read Callback"="", "Write Callback"="rsscope_FormatSearchNameEvent_WriteCallback.vi", "Supported Models"="", "Instrument Options"="", "Flags"=0, "Help"="Copies the trigger event configuration from Trigger A for the selected channel source to the search condition settings. Set the selected search name with RSSCOPE_ATTR_SELECTED_SEARCH_NAME.\n\nAvailable Repeated Capabilities:\nNone\n\nRemote-control command(s):\nSEARch:TRIGger:SETHold:ACOPy"}, {"Level"=3, "Class Only"=TRUE, "Identifier"="", "Descriptive Name"="State", "Data Type"=0, "Command"="", "Access"=0, "Range Table"="", "Read Callback"="", "Write Callback"="", "Supported Models"="", "Instrument Options"="", "Flags"=0, "Help"="This function configures the conditions for the state 
